vi "tarea1.vi"() -> ()   [LabVIEW 2016]
panel:
  in  "c":dbl
  in  "b":dbl
  out "x2":dbl
  out "x1":dbl
  in  "a":dbl
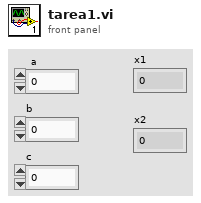
[diagram p1: front panel]
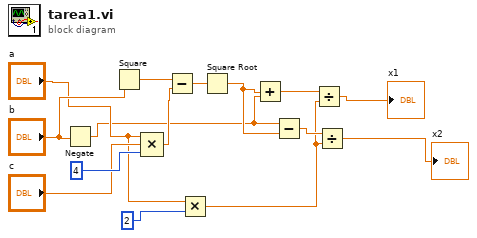
[diagram p0: block diagram]
diagram:
  n1 = Negate(x="b") -> (-x=w1:dbl)
  n2 = Square(x="b") -> (x^2=w14:dbl)
  n3 = Compound Arithmetic op=MULTIPLY("a", "c", 4) -> (w13:dbl)
  n4 = Subtract(x=w14, y=w13) -> (x-y=w12:dbl)
  n5 = Multiply(x="a", y=2) -> (x*y=w6:dbl)
  n6 = Square Root(x=w12) -> (sqrt(x)=w4:dbl)
  n7 = Add(x=w4, y=w1) -> (x+y=w7:dbl)
  n8 = Subtract(x=w1, y=w4) -> (x-y=w8:dbl)
  n9 = Divide(x=w7, y=w6) -> (x/y=→"x1":dbl)
  n10 = Divide(x=w8, y=w6) -> (x/y=→"x2":dbl)
